vi "ConcatenateOntoShortcutMenu.vi"(8 "error in":errorcluster, 9 "menu ref in":refnum<k9>, 11 "Thermo in":refnum<class "Thermo Instrument.lvclass">) -> (0 "error out":errorcluster, 1 "menu ref out":refnum<k9>, 3 "Thermo out":refnum<class "Thermo Instrument.lvclass">)   [LabVIEW 2025, in "Thermo.lvlib" / "Thermo Instrument.lvclass"]
doc: "Allows children to insert menu items without overriding ShortcutMenu.vi entirely. By default, called after Add/Remove.Copyright 2017 National Instruments Corporation\n\nLicensed under the Apache License, Version 2.0 (the \"License\"); you may not use this file except in compliance with the License. You may obtain a copy of the License at http://www.apache.org/licenses/LICENSE-2.0\nUnless required by applicable law or agreed to in writing, software distributed under the License is distributed on an \"AS IS\" BASIS, WITHOUT WARRANTIES OR CONDITIONS OF ANY KIND, either express or implied. See the License for the specific language governing permissions and limitations under the License."
uses:
  Thermo Instrument.lvclass
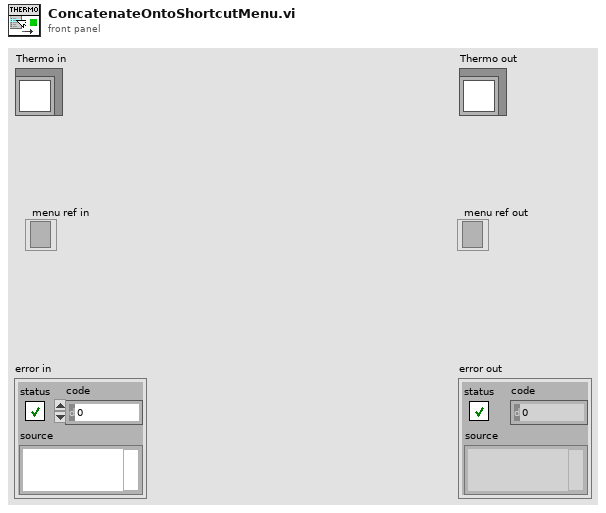
[diagram p1: front panel]
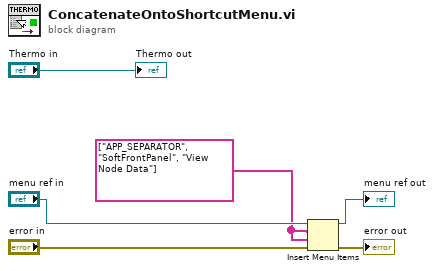
[diagram p0: block diagram]
diagram:
  w1 = string[] ["APP_SEPARATOR", "SoftFrontPanel", "View Node Data"]
  n1 = Insert Menu Items(6:"error in", 7:w1, 8:w1, 9:"menu ref in") -> (0:→"error out":errorcluster, 3:→"menu ref out":refnum<k9>)  [unwired: 2 in, 1 out]
  "Thermo out" <- "Thermo in"
